vi "OEE_save_database_password.vi"(7 "error_in":errorcluster, 9 "new_password":string, 10 "all_config_info_in":T1={"main_ini_file"={"SQL Driver"="", "SQL Server"="", "SQL Database"="", "SQL UID"="", "Reference table"="", "Reference history"="", "Archivisation CFG table"="", "Archivisation CFG history"="", "User table"="", "User history"="", "Default reference"="", "Update pulse[ms]"=0, "default language"="", "SCREEN 1 Left"=10, "SCREEN 1 Top"=0, "SCREEN 1 Width"=0, "SCREEN 1 Height"=0, "SCREEN 2 Left"=0, "SCREEN 2 Top"=0, "SCREEN 2 Width"=0, "SCREEN 2 Height"=10}, "SQL Password"="", "queue_refnums"={"MAIN_queue"=refnum, "SCREEN_1_queue"=refnum, "SCREEN_2_queue"=refnum, "PULSE_queue"=refnum, "GRAPH_TOGGLE_queue"=refnum}}) -> (0 "error_out":errorcluster, 3 "all_config_info_out":T1={"main_ini_file"={"SQL Driver"="", "SQL Server"="", "SQL Database"="", "SQL UID"="", "Reference table"="", "Reference history"="", "Archivisation CFG table"="", "Archivisation CFG history"="", "User table"="", "User history"="", "Default reference"="", "Update pulse[ms]"=0, "default language"="", "SCREEN 1 Left"=10, "SCREEN 1 Top"=0, "SCREEN 1 Width"=0, "SCREEN 1 Height"=0, "SCREEN 2 Left"=0, "SCREEN 2 Top"=0, "SCREEN 2 Width"=0, "SCREEN 2 Height"=10}, "SQL Password"="", "queue_refnums"={"MAIN_queue"=refnum, "SCREEN_1_queue"=refnum, "SCREEN_2_queue"=refnum, "PULSE_queue"=refnum, "GRAPH_TOGGLE_queue"=refnum}})   [LabVIEW 2019]
uses:
  ini/typedef/OEE_all_config_info.ctl
  ini/typedef/OEE_main_ini_file.ctl
  queues/typedef/OEE_queue_refnums.ctl
  queues/typedef/OEE_MAIN_queue_element.ctl
  MAIN/OEE_MAIN_sequence_state.ctl
  queues/typedef/OEE_SCREEN_1_queue_element.ctl
  SCREEN_1/OEE_SCREEN_1_sequence_state.ctl
  queues/typedef/OEE_SCREEN_2_queue_element.ctl
  SCREEN_2/OEE_SCREEN_2_sequence_state.ctl
  queues/typedef/OEE_PULSE_queue_element.ctl
  PULSE/OEE_PULSE_sequence_state.ctl
  queues/typedef/OEE_GRAPH_TOGGLE_TIMER_queue_element.ctl
  SCREEN_2/GRAPH_TOGGLE_TIMER/OEE_GRAPH_TOGGLE_TIMER_sequence_state.ctl
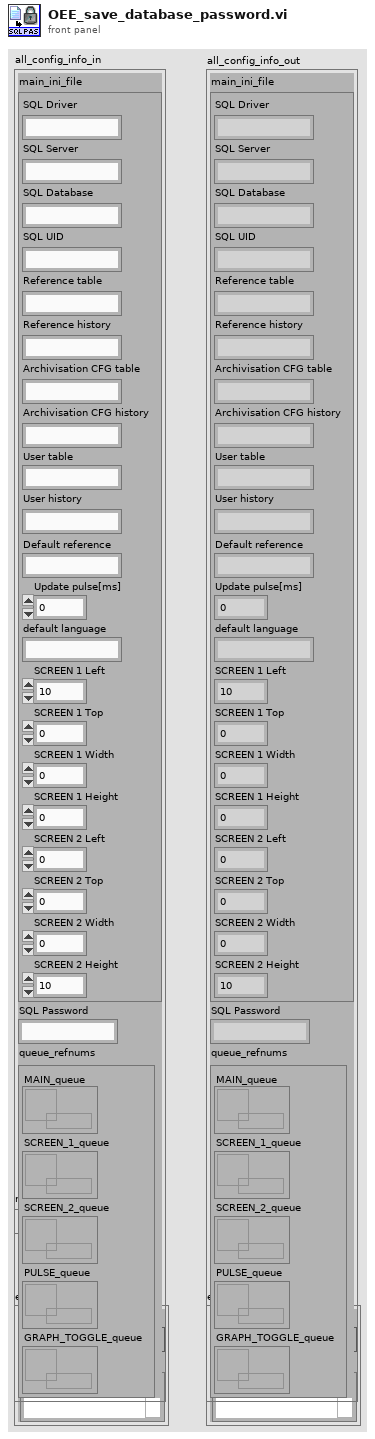
[diagram p1: front panel]
types:
  T1 = typedef "OEE_all_config_info.ctl" = cluster{"main_ini_file":T2, "SQL Password":string, "queue_refnums":T3}
  T2 = typedef "OEE_main_ini_file.ctl" = cluster{"SQL Driver":string, "SQL Server":string, "SQL Database":string, "SQL UID":string, "Reference table":string, "Reference history":string, "Archivisation CFG table":string, "Archivisation CFG history":string, "User table":string, "User history":string, "Default reference":string, "Update pulse[ms]":i32, "default language":string, "SCREEN 1 Left":i16, "SCREEN 1 Top":i16, "SCREEN 1 Width":i16, "SCREEN 1 Height":i16, "SCREEN 2 Left":i16, "SCREEN 2 Top":i16, "SCREEN 2 Width":i16, "SCREEN 2 Height":i16}
  T3 = typedef "OEE_queue_refnums.ctl" = cluster{"MAIN_queue":refnum<queue>, "SCREEN_1_queue":refnum<queue>, "SCREEN_2_queue":refnum<queue>, "PULSE_queue":refnum<queue>, "GRAPH_TOGGLE_queue":refnum<queue>}
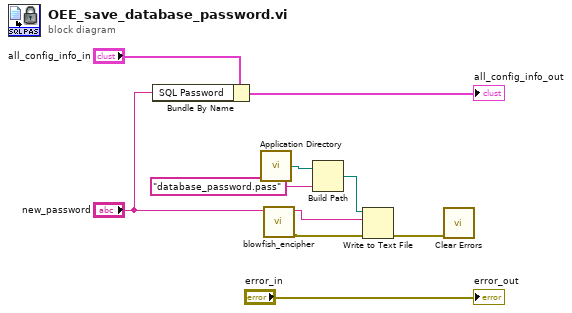
[diagram p0: block diagram]
diagram:
  n1 = Bundle By Name(cluster="all_config_info_in", "SQL Password"="new_password") -> (→"all_config_info_out":T1)
  n2 = call <vilib>:"Application Directory.vi"() -> ("Application Directory"=w9:path)
  n3 = call "blowfish_encipher.vi"("Input Text"="new_password") -> ("error out"=w5:errorcluster, "Output Text"=w4:string)  [unwired: 9 in]
  n4 = Build Path(base path=w9, name or relative path="database_password.pass") -> (appended path=w7:path)
  n5 = Write to Text File(file (use dialog)=w7, text=w4, error in=w5) -> (error out=w6:errorcluster)  [unwired: 1 in, 2 out]
  n6 = call <vilib>:"Clear Errors.vi"("error in (no error)"=w6) -> ()  [unwired: 5 in, 2 out]
  "error_out" <- "error_in"
